vi "Polarisation_v2.vi"(0 "Test Handles Polar":T5, 1 "Polar Params SubVIv2":T2, 3 "Test References":T6) -> (4 "2D Pol Data":dbl[][](array[numeric]), 5 "Test Handles Out":T4, 6 "Angles":dbl[](array[numeric]), 7 "Wavelengths":dbl[](array[numeric]), 8 "Puissances":dbl[](array[numeric]))   [LabVIEW 2019]
uses:
  Light Field/lightfield-automation-labview/LightField Automation.lvclass
  TypeDefs/AcqMode.ctl
  C:/Users/manip/Documents/Controle_Manip_2020/Thorlabs.MotionControl.KCube.SolenoidCLI.dll
  Thorlabs.MotionControl.KCube.SolenoidCLI.dll
  Newport/Newport ESP301/Newport ESP301.lvlib
panel:
  out "Photodiode error out":errorcluster
  out "Photodiode handle out":refnum<visa-resource-name>
  in  "Polar Params SubVI 2":T3
  out "Shutter on?":bool
  in  "Polar mode":u16(ring)=3 caption="Rotate HWP" items=["Excitation"=3, "Detection"=2]
  out "KCube Shutter Device Reference":refnum<k24>
  in  "Previous Button":bool
  in  "StopPolar":bool
  out "CCD 1D Spectrum Main 2":cluster{dbl[], dbl[]}(graph)
  in  "XYGraph Refnum":refnum<vi>
  in  "Acq Mode":T1=enum."Spectrum" caption="Acq mode"
  out "2D Data":dbl[][](array[numeric])
  in  "RotStage Exc Angle (°)":dbl=2.0 caption="Readout (°)" min=-360.0 max=360.0
  out "Position (units)":dbl format="%.6g"
  out "Numeric":i32
  out "Motion Done":bool
  in  "Progress":u8(slide) scale=0.0..100.0
  out "Current angle (°)":dbl
  in  "CCD ROI":T7(ring)
  out "ESP301 Error out":errorcluster
  out "LightField error out":errorcluster
  out "ESP301 Error":errorcluster
  in  "Exposure time (ms)":dbl=100.0
  in  "Axis ESP301 / RotStage":u16(ring) items=["RotStage Detection"=2, "RotStage Excitation"=3]
  in  "Step Angle (°)":dbl=5.0
  in  "End Angle (°)":dbl=180.0
  in  "Start Angle (°)":dbl
  out "LightField Automation out":refnum<class "LightField Automation.lvclass">
  out "VISA resource name out":refnum<visa-resource-name>
types:
  T1 = typedef "AcqMode.ctl" = enum16{"Image", "Spectrum", "APD 1", "APD 2", "APD 1+2"}
  T2 = cluster{"Polar End Angle (°)":dbl, "Polar Start Angle (°)":dbl, "Polar Step Angle (°)":dbl, "Acq Mode":T1, "Polar mode":u16, "Exposure Time (ms)":dbl, "CCD ROI":enum16{"Custom ROI", "Full sensor", "Binned full sensor"}, "KCube Shutter On?":bool}
  T3 = cluster{"Polar End Angle (°)":dbl, "Polar Start Angle (°)":dbl, "Polar Step Angle (°)":dbl, "Acq Mode":T1, "Polar mode":u16, "Exposure Time (ms)":dbl, "CCD ROI":enum16{"Custom ROI", "Full sensor", "Binned full sensor"}}
  T4 = cluster{"LightField Automation out":refnum<class "LightField Automation.lvclass">, "LightField error out":errorcluster, "VISA resource name out":refnum<visa-resource-name>, "ESP301 Error":errorcluster, "Photodiode handle out":refnum<visa-resource-name>, "Photodiode error out":errorcluster}
  T5 = cluster{"LightField Automation out":refnum<class "LightField Automation.lvclass">, "LightField Automation error out":errorcluster, "ESP 301 COM Port":refnum<visa-resource-name>, "ESP 301 Error":errorcluster, "Photodiode handle out":refnum<visa-resource-name>, "Photodiode error out":errorcluster}
  T6 = cluster{"Acquire Polarisation":refnum<vi>, "Save Polarisation":refnum<vi>, "PausePolar":refnum<vi>, "StopPolar":refnum<vi>, "Scan Main Progess Bar":refnum<vi>, "RotStage Exc Angle Readout (°)":refnum<vi>, "RotStage Det Angle Readout (°)":refnum<vi>, "Polarisation 1D Spectrum":refnum<vi>, "Polarisation 2D Image":refnum<vi>, "Shutter Ctrls":refnum<vi>, "KCube Shutter Device Reference":refnum<vi>}
  T7 = enum16{"Custom ROI", "Full sensor", "Binned full sensor"}
  T8 = enum16{"Contrast", "Spectre", "Polarisation", "Time Trace", "XY Intensity Map"}
  T9 = cluster{"Image":dbl[][][], "Frame Size":cluster{"F":i32, "Y":i32, "X":i32}}[]
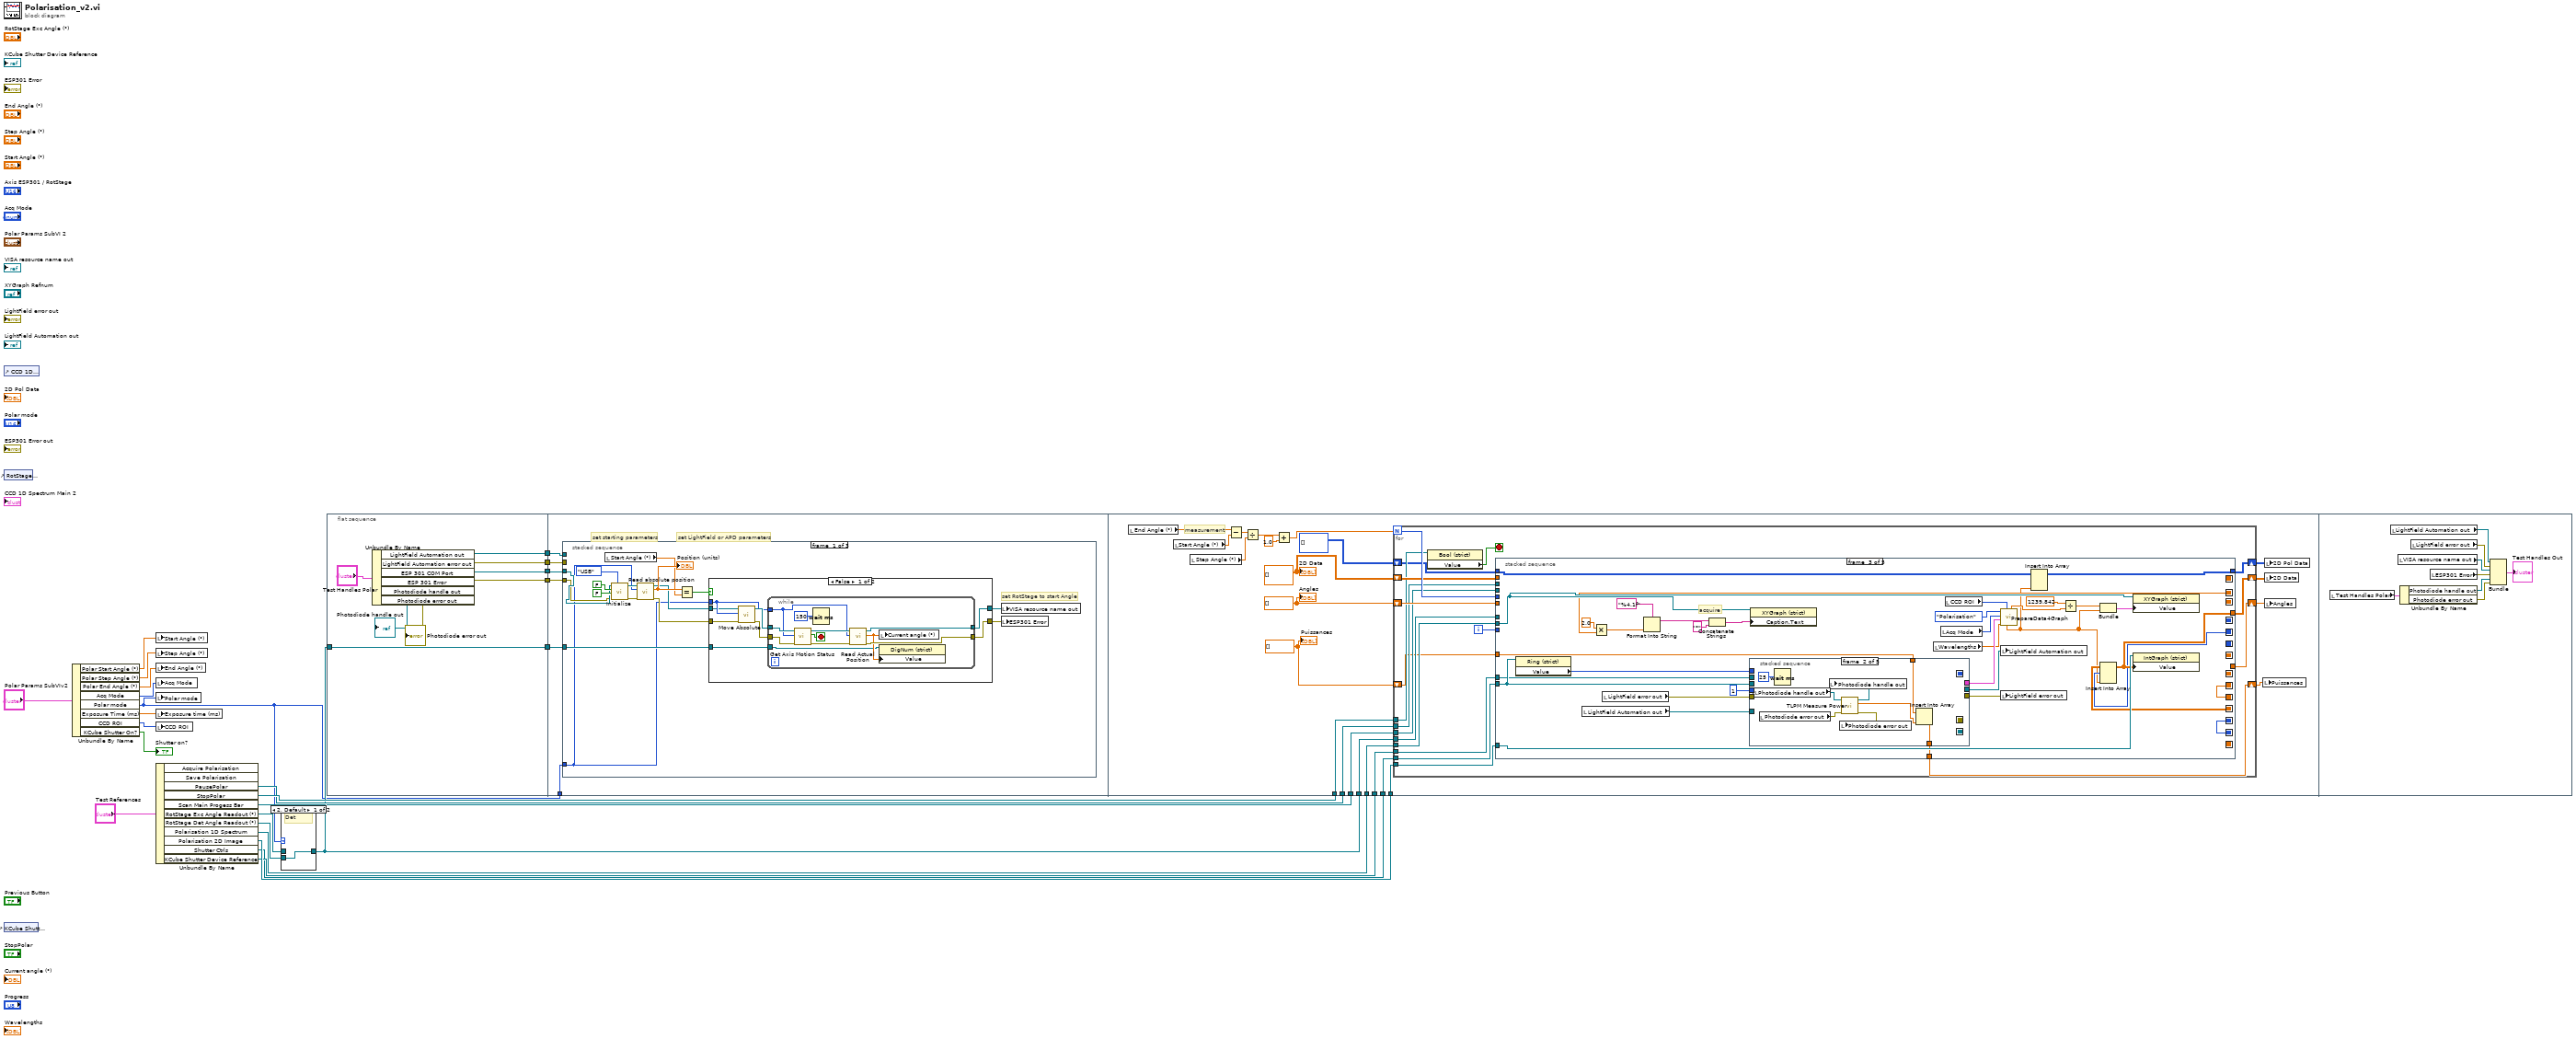
[diagram p0: block diagram]
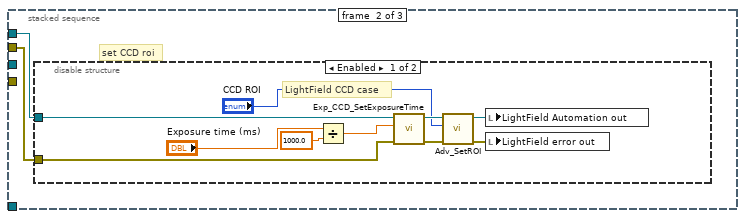
[diagram p4: hidden frame]
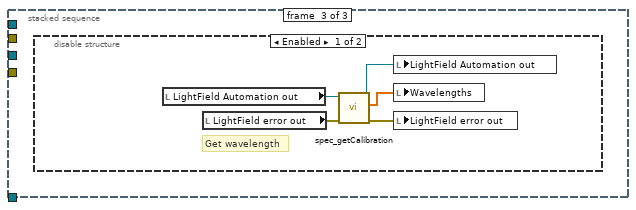
[diagram p6: hidden frame]
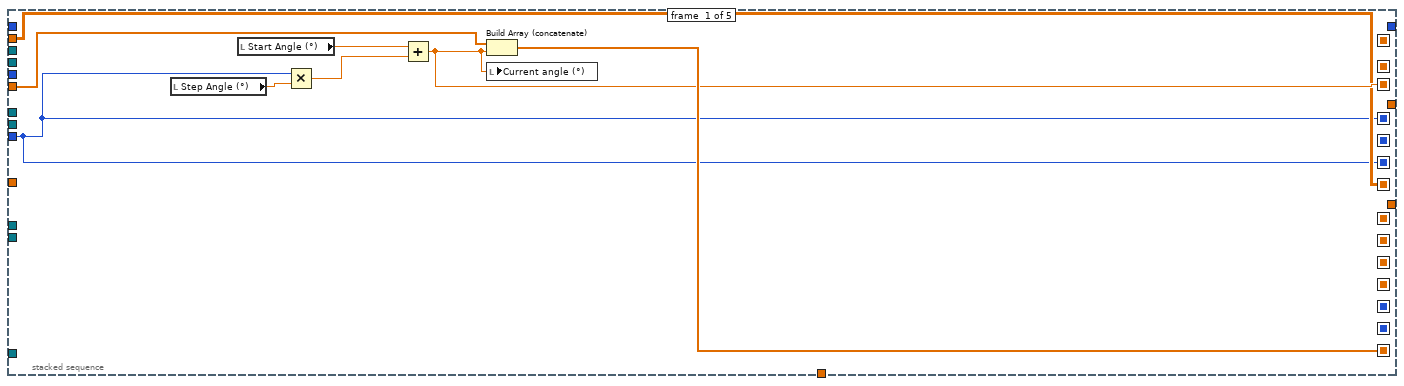
[diagram p8: hidden frame]
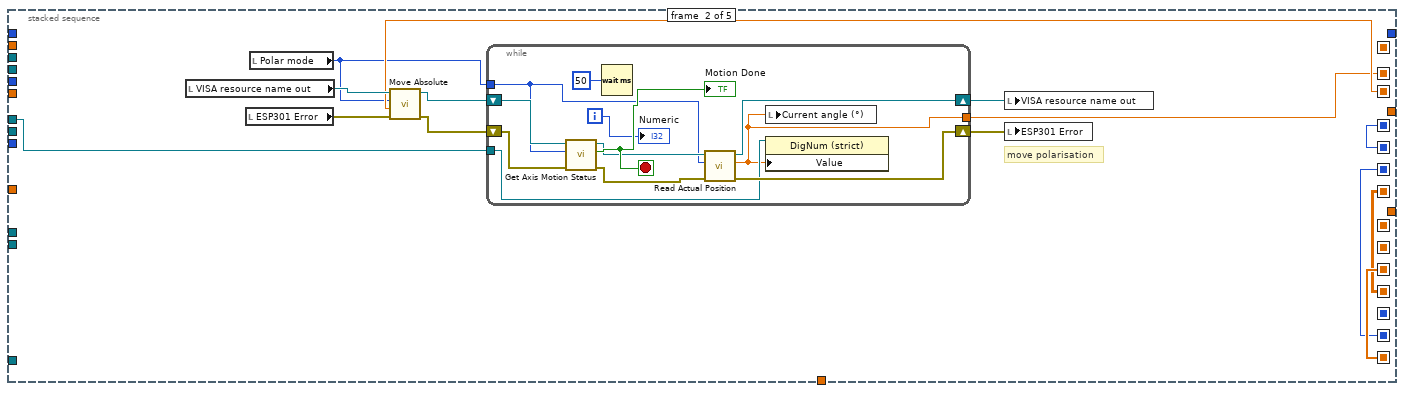
[diagram p9: hidden frame]
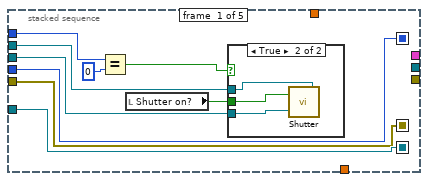
[diagram p10: hidden frame]
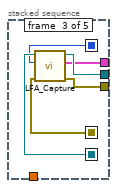
[diagram p12: hidden frame]
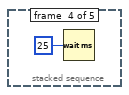
[diagram p13: hidden frame]
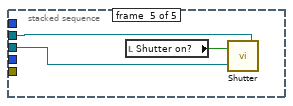
[diagram p14: hidden frame]
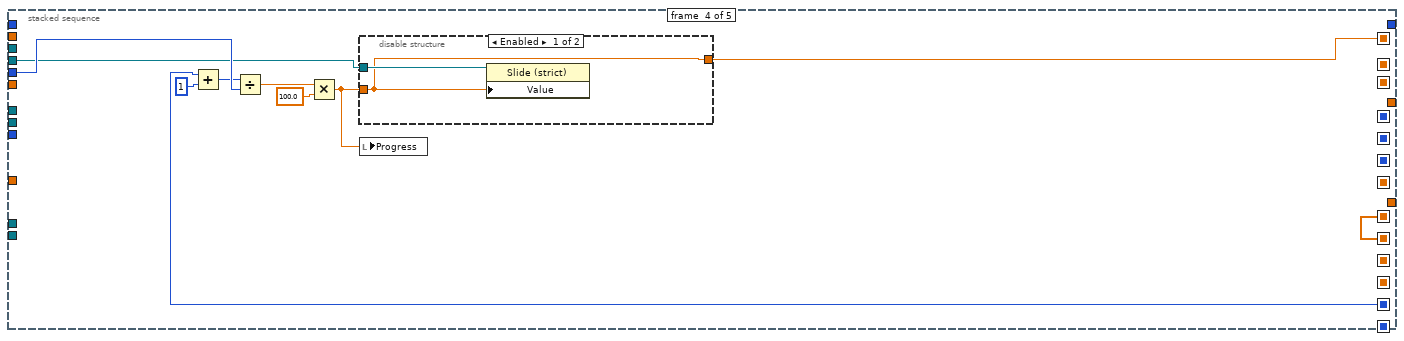
[diagram p15: hidden frame]
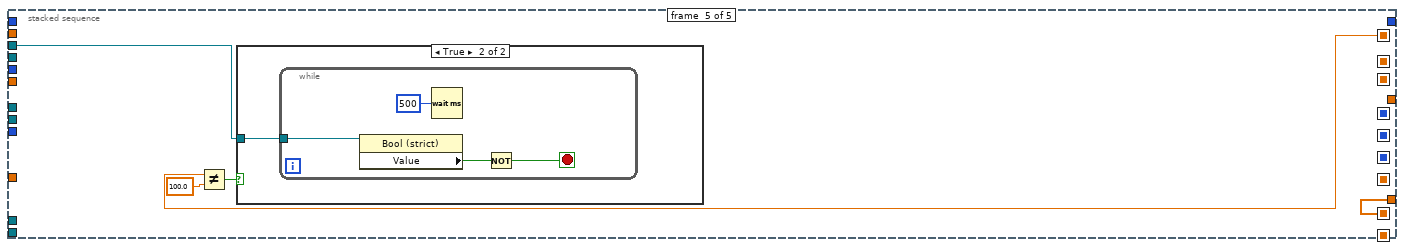
[diagram p17: hidden frame]
diagram:
  n1 = control-ref of="CCD 1D Spectrum Main 2"() -> ()  [unwired: 1 out]
  n2 = control-ref of="RotStage Exc Angle (°)"() -> ()  [unwired: 1 out]
  n3 = control-ref of="KCube Shutter Device Reference"() -> ()  [unwired: 1 out]
  n4 = Unbundle By Name("Polar Params SubVIv2") -> ("Polar Start Angle (°)"=w7:dbl, "Polar Step Angle (°)"=w6:dbl, "Polar End Angle (°)"=w5:dbl, "Acq Mode"=w4:T1, "Polar mode"=w8:u16, "Exposure Time (ms)"=w3:dbl, "CCD ROI"=w2:T7, "KCube Shutter On?"=→"Shutter on?":bool)
  n5 = local write "Start Angle (°)"(w7) -> ()
  n6 = local write "Step Angle (°)"(w6) -> ()
  n7 = local write "End Angle (°)"(w5) -> ()
  n8 = local write "Acq Mode"(w4) -> ()
  n9 = local write "Polar mode"(w8) -> ()
  n10 = local write "Exposure time (ms)"(w3) -> ()
  n11 = local write "CCD ROI"(w2) -> ()
  n12 = Unbundle By Name("Test References") -> ("PausePolar"=w23:refnum<vi>, "StopPolar"=w24:refnum<vi>, "Scan Main Progess Bar"=w17:refnum<vi>, "RotStage Exc Angle Readout (°)"=w18:refnum<vi>, "RotStage Det Angle Readout (°)"=w19:refnum<vi>, "Polarisation 1D Spectrum"=w22:refnum<vi>, "Polarisation 2D Image"=w21:refnum<vi>, "Shutter Ctrls"=w14:refnum<vi>, "KCube Shutter Device Reference"=w15:refnum<vi>)  [unwired: 2 out]
  n13 = case shown="2, Default" w8 {
    tunnel: [w26 w27] -> w20
    tunnel: w19 -> [w26 _]
    tunnel: w18 -> [_ w27]
    frame 2, Default {
      # "Det"
    }
    frame 3 {
      # "Exc"
    }
  }
  n14 = flat-sequence {
    tunnel: w20 -> [w35]
    tunnel: [w35] -> w25
    tunnel: [w33] -> w13
    tunnel: [w32] -> w12
    tunnel: [w31] -> w11
    tunnel: [w30] -> w10
    tunnel: w25 -> [w41]
    tunnel: w13 -> [w40]
    tunnel: w12 -> [w39]
    tunnel: w11 -> [w38]
    tunnel: w10 -> [w37]
    tunnel: w8 -> [w36]
    tunnel: w20 -> [w109]
    tunnel: w21 -> [w108]
    tunnel: w22 -> [w105]
    tunnel: w24 -> [w104]
    tunnel: w23 -> [w103]
    tunnel: w17 -> [w100]
    tunnel: w14 -> [w99]
    tunnel: w15 -> [w98]
    frame #0 {
      n15 = Unbundle By Name("Test Handles Polar") -> ("LightField Automation out"=w31:refnum<class "LightField Automation.lvclass">, "LightField Automation error out"=w30:errorcluster, "ESP 301 COM Port"=w33:refnum<visa-resource-name>, "ESP 301 Error"=w32:errorcluster, "Photodiode handle out"=→"Photodiode handle out":refnum<visa-resource-name>, "Photodiode error out"=→"Photodiode error out":errorcluster)
    }
    frame #1 {
      # "set LightField or APD parameters"
      # "set starting parameters"
      n16 = stacked-sequence {
        tunnel: w41 -> [w45 _ _]
        tunnel: w40 -> [w44 _ _]
        tunnel: w39 -> [w43 _ _]
        tunnel: w38 -> [_ w80 _]
        tunnel: w37 -> [_ w79 _]
        tunnel: w36 -> [w42 _ _]
        frame #0 {
          # "set RotStage to start Angle"
          n17 = local read "Start Angle (°)"() -> (w54:dbl)
          n18 = call "Initialize.vi"("VISA resource name"=w44, "ID Query (True)"=FALSE, "Reset (False)"=FALSE, "error in (no error)"=w43, "Serial Link (RS232)"=enum16{"RS232", "USB"}."USB") -> ("VISA resource name out"=w47:refnum<visa-resource-name>, "error out"=w46:errorcluster)  [unwired: 4 in]
          n19 = call "Read absolute position.vi"("error in (no error)"=w46, "Axis (1)"=w42, "VISA resource name"=w47) -> ("error out"=w52:errorcluster, "Position (units)"=w55:dbl, "VISA resource name out"=w51:refnum<visa-resource-name>)  [unwired: 2 in]
          "Position (units)" <- w55
          n20 = Equal?(x=w55, y=w54) -> (x = y?=w53:bool)
          n21 = case shown="False" w53 {
            tunnel: [w65 w78] -> w57
            tunnel: [w64 w77] -> w56
            tunnel: w42 -> [w61 _]
            tunnel: w52 -> [w60 w77]
            tunnel: w51 -> [w59 w78]
            tunnel: w45 -> [w58 _]
            frame False {
              n22 = call "Move Absolute.vi"("error in (no error)"=w60, "Axis (1)"=w61, "VISA resource name"=w59) -> ("error out"=w62:errorcluster, "VISA resource name out"=w63:refnum<visa-resource-name>)  [unwired: 3 in]
              n23 = while {
                tunnel: w61 -> [w70]
                tunnel: w58 -> [w66]
                tunnel: w63 -> [w76]
                tunnel: [w71] -> w65
                tunnel: w62 -> [w75]
                tunnel: [w68] -> w64
                stop <- w74 stop-if-true
                n24 = call "Get Axis Motion Status.vi"("error in (no error)"=w75, "Axis (1)"=w70, "VISA resource name"=w76) -> ("error out"=w69:errorcluster, "Motion Done"=w74:bool, "VISA resource name out"=w72:refnum<visa-resource-name>)  [unwired: 2 in]
                n25 = Wait (ms)(milliseconds to wait=u32 150) -> ()  [unwired: 1 out]
                n26 = call "Read Actual Position.vi"("error in (no error)"=w69, "Axis (1)"=w70, "VISA resource name"=w72) -> ("error out"=w68:errorcluster, "Position (units)"=w67:dbl, "VISA resource name out"=w71:refnum<visa-resource-name>)  [unwired: 2 in]
                n27 = local write "Current angle (°)"(w67) -> ()
                n28 = property class="DigNum (strict)"(reference=w66, "Value"=w67) -> ()  [unwired: 1 in, 2 out]
              }
            }
            frame True {
            }
          }
          n29 = local write "VISA resource name out"(w57) -> ()
          n30 = local write "ESP301 Error"(w56) -> ()
        }
        frame #1 {
          # "set CCD roi"
          n31 = disable-structure shown="Enabled" {
            disable-tunnel: w80 -> [w82 _]
            disable-tunnel: w79 -> [w81 _]
            frame Enabled {
              # "LightField CCD case"
              n32 = Divide(x="Exposure time (ms)", y=1000.0) -> (x/y=w88:dbl)
              n33 = call "Exp_CCD_SetExposureTime.vi"("error in (no error)"=w81, "Exposure Time (s)"=w88, "LightField Automation in"=w82) -> ("error out"=w86:errorcluster, "LightField Automation out"=w87:refnum<class "LightField Automation.lvclass">)  [unwired: 7 in]
              n34 = call "Adv_SetROI.vi"("error in (no error)"=w86, "ROI"="CCD ROI", "LightField Automation in"=w87) -> ("error out"=w85:errorcluster, "LightField Automation out"=w84:refnum<class "LightField Automation.lvclass">)  [unwired: 7 in]
              n35 = local write "LightField Automation out"(w84) -> ()
              n36 = local write "LightField error out"(w85) -> ()
            }
            frame Disabled {
            }
          }
        }
        frame #2 {
          n37 = disable-structure shown="Enabled" {
            frame Enabled {
              # "Get wavelength"
              n38 = local read "LightField Automation out"() -> (w95:refnum<class "LightField Automation.lvclass">)
              n39 = local read "LightField error out"() -> (w94:errorcluster)
              n40 = call "spec_getCalibration.vi"("error in (no error)"=w94, "LightField Automation in"=w95) -> ("error out"=w92:errorcluster, "ColumnCalibration"=w91:dbl[], "LightField Automation out"=w93:refnum<class "LightField Automation.lvclass">)  [unwired: 7 in]
              n41 = local write "LightField Automation out"(w93) -> ()
              n42 = local write "Wavelengths"(w91) -> ()
              n43 = local write "LightField error out"(w92) -> ()
            }
            frame Disabled {
            }
          }
        }
      }
    }
    frame #2 {
      w97 = dbl[] []
      w107 = dbl[][] []
      w110 = dbl[] []
      # "measurement"
      n44 = local read "End Angle (°)"() -> (w112:dbl)
      n45 = local read "Start Angle (°)"() -> (w113:dbl)
      n46 = local read "Step Angle (°)"() -> (w115:dbl)
      n47 = Subtract(x=w112, y=w113) -> (x-y=w114:dbl)
      n48 = Divide(x=w114, y=w115) -> (x/y=w116:dbl)
      n49 = Add(x=w116, y=1.0) -> (x+y=w117:dbl)
      n50 = for {
        N: w117 -> [w134]
        shift-right: [w136] -> w118
        shift-left: w110 -> [w137]
        tunnel: w100 -> [w133]
        tunnel: w109 -> [w132]
        tunnel: w108 -> [w131]
        shift-right: [w129] -> w106
        shift-left: w107 -> [w130]
        tunnel: w105 -> [w128]
        tunnel: w104 -> [w127]
        tunnel: w103 -> [w125]
        shift-right: [w123] -> w101
        shift-left: i32[][] [] -> [w124]
        tunnel: w99 -> [w122]
        tunnel: w98 -> [w121]
        shift-right: [w119] -> w96
        shift-left: w97 -> [w120]
        i -> [w135]
        stop <- w126 stop-if-true
        n51 = property class="Bool (strict)"(reference=w127) -> ("Value"=w126:bool)  [unwired: 1 in, 2 out]
        n52 = stacked-sequence {
          seq-local: [w144 _ _ _ _] -> [_ w159 _ _ _]
          seq-local: [w138 _ _ _ _] -> [_ w158 _ _ _]
          seq-local: [w140 _ _ _ _] -> [_ w155 _ _ _]
          seq-local: [w139 _ _ _ _] -> [_ w148 _ _ _]
          seq-local: [w138 _ _ _ _] -> [_ w147 _ _ _]
          seq-local: [_ w159 _ _ _] -> [_ _ w204 _ _]
          seq-local: [_ w158 _ _ _] -> [_ _ w207 _ _]
          seq-local: [_ w148 _ _ _] -> [_ _ w205 _ _]
          seq-local: [_ w147 _ _ _] -> [_ _ w202 _ _]
          seq-local: [_ w146 _ _ _] -> [_ _ w183 _ _]
          seq-local: [_ _ w204 _ _] -> [_ _ _ w247 _]
          seq-local: [_ _ w207 _ _] -> [_ _ _ w243 _]
          seq-local: [_ _ _ w247 _] -> [_ _ _ _ w254]
          seq-local: [_ _ _ w238 _] -> [_ _ _ _ w252]
          tunnel: w137 -> [w145 _ _ _ _]
          tunnel: w135 -> [w138 _ _ _ _]
          tunnel: w130 -> [w139 _ _ _ _]
          tunnel: w132 -> [_ w149 _ _ _]
          tunnel: w131 -> [_ _ w206 _ _]
          tunnel: [_ _ w203 _ _] -> w129
          tunnel: w128 -> [_ _ w193 _ _]
          tunnel: w124 -> [_ _ w181 _ _]
          tunnel: [_ _ w180 _ _] -> w123
          tunnel: w122 -> [_ _ w175 _ _]
          tunnel: w121 -> [_ _ w174 _ _]
          tunnel: w134 -> [_ _ _ w244 _]
          tunnel: w133 -> [_ _ _ w240 _]
          tunnel: [_ _ _ _ w254] -> w136
          tunnel: w125 -> [_ _ _ _ w253]
          tunnel: w120 -> [_ _ w173 _ _]
          tunnel: [_ _ w172 _ _] -> w119
          frame #0 {
            n53 = local read "Step Angle (°)"() -> (w142:dbl)
            n54 = local read "Start Angle (°)"() -> (w143:dbl)
            n55 = Multiply(x=w138, y=w142) -> (x*y=w141:dbl)
            n56 = Add(x=w143, y=w141) -> (x+y=w140:dbl)
            n57 = Build Array (concatenate)(w145, w140) -> (w144:dbl[])
            n58 = local write "Current angle (°)"(w140) -> ()
          }
          frame #1 {
            # "move polarisation"
            n59 = local read "VISA resource name out"() -> (w157:refnum<visa-resource-name>)
            n60 = local read "ESP301 Error"() -> (w156:errorcluster)
            n61 = local read "Polar mode"() -> (w152:u16)
            n62 = call "Move Absolute.vi"("error in (no error)"=w156, "Position (0 units)"=w155, "Axis (1)"=w152, "VISA resource name"=w157) -> ("error out"=w154:errorcluster, "VISA resource name out"=w153:refnum<visa-resource-name>)  [unwired: 2 in]
            n63 = while {
              tunnel: w152 -> [w164]
              shift-right: [w163] -> w150
              shift-left: w153 -> [w169]
              shift-right: [w162] -> w151
              shift-left: w154 -> [w170]
              tunnel: w149 -> [w161]
              tunnel: [w160] -> w146
              i -> [w168]
              stop <- w171 stop-if-true
              n64 = call "Get Axis Motion Status.vi"("error in (no error)"=w170, "Axis (1)"=w164, "VISA resource name"=w169) -> ("error out"=w166:errorcluster, "Motion Done"=w171:bool, "VISA resource name out"=w165:refnum<visa-resource-name>)  [unwired: 2 in]
              "Motion Done" <- w171
              n65 = Wait (ms)(milliseconds to wait=u32 50) -> ()  [unwired: 1 out]
              n66 = call "Read Actual Position.vi"("error in (no error)"=w166, "Axis (1)"=w164, "VISA resource name"=w165) -> ("error out"=w162:errorcluster, "Position (units)"=w160:dbl, "VISA resource name out"=w163:refnum<visa-resource-name>)  [unwired: 2 in]
              n67 = local write "Current angle (°)"(w160) -> ()
              n68 = property class="DigNum (strict)"(reference=w161, "Value"=w160) -> ()  [unwired: 1 in, 2 out]
              "Numeric" <- w168
            }
            n69 = local write "VISA resource name out"(w150) -> ()
            n70 = local write "ESP301 Error"(w151) -> ()
          }
          frame #2 {
            # "acquire"
            n71 = property class="Ring (strict)"(reference=w175) -> ("Value"=w182:u16)  [unwired: 1 in, 2 out]
            n72 = local read "LightField Automation out"() -> (w201:refnum<class "LightField Automation.lvclass">)
            n73 = Multiply(x=2.0, y=w183) -> (x*y=w185:dbl)
            n74 = local read "LightField error out"() -> (w200:errorcluster)
            n75 = Format Into String(format string="%4.1f", w185) -> (resulting string=w192:string)  [unwired: 2 in, 1 out]
            n76 = Concatenate Strings(w192, "°") -> (w190:string)
            n77 = stacked-sequence {
              seq-local: [w216 _ _ _ _] -> [_ _ w233 _ _]
              seq-local: [w215 _ _ _ _] -> [_ _ w232 _ _]
              seq-local: [w214 _ _ _ _] -> [_ _ w228 _ _]
              tunnel: w201 -> [w216 _ _ _ _]
              tunnel: w200 -> [w215 _ _ _ _]
              tunnel: 1 ("Frames") -> [w214 _ _ _ _]
              tunnel: [_ _ w231 _ _] -> w199
              tunnel: [_ _ w230 _ _] -> w198
              tunnel: [_ _ w229 _ _] -> w197
              tunnel: w175 -> [w212 _ _ _ w237]
              tunnel: w174 -> [w213 _ _ _ w236]
              tunnel: w182 -> [w211 _ _ _ _]
              tunnel: w173 -> [_ w222 _ _ _]
              tunnel: [_ w220 _ _ _] -> w172
              frame #0 {
                n78 = Equal?(x=w211, y=u16 0) -> (x = y?=w210:bool)
                n79 = local read "Shutter on?"() -> (w208:bool)
                n80 = case shown="True" w210 {
                  tunnel: w213 -> [_ w219]
                  tunnel: w212 -> [_ w218]
                  tunnel: w208 -> [_ w217]
                  frame False {
                  }
                  frame True {
                    n81 = call "Shutter.vi"("KCube Shutter Device Reference 2"=w219, "Shutter Ctrls 2"=w218, "Shutter on?"=w217) -> ()
                  }
                }
              }
              frame #1 {
                n82 = local read "Photodiode handle out"() -> (w226:refnum<visa-resource-name>)
                n83 = local read "Photodiode error out"() -> (w225:errorcluster)
                n84 = Wait (ms)(milliseconds to wait=u32 25) -> ()  [unwired: 1 out]
                n85 = call <instrlib>:"TLPM Measure Power.vi"("error in (no error)"=w225, "instrument handle"=w226) -> ("error out"=w223:errorcluster, "Power"=w221:dbl, "instrument handle out"=w224:refnum<visa-resource-name>)  [unwired: 7 in]
                n86 = local write "Photodiode handle out"(w224) -> ()
                n87 = local write "Photodiode error out"(w223) -> ()
                n88 = Insert Into Array(array=w222, new element=w221) -> (w220:dbl[])  [unwired: 1 in]
              }
              frame #2 {
                n89 = call "LFA_Capture.vi"("error in (no error)"=w232, "Frames"=w228, "LightField Automation in"=w233) -> ("error out"=w231:errorcluster, "Data"=w229:T9, "LightField Automation out"=w230:refnum<class "LightField Automation.lvclass">)  [unwired: 6 in]
              }
              frame #3 {
                n90 = Wait (ms)(milliseconds to wait=u32 25) -> ()  [unwired: 1 out]
              }
              frame #4 {
                n91 = local read "Shutter on?"() -> (w235:bool)
                n92 = call "Shutter.vi"("KCube Shutter Device Reference 2"=w236, "Shutter Ctrls 2"=w237, "Shutter on?"=w235) -> ()
              }
            }
            n93 = property class="XYGraph (strict)"(reference=w193, "Caption.Text"=w190) -> ()  [unwired: 1 in, 2 out]
            n94 = local read "Wavelengths"() -> (w194:dbl[])
            n95 = local read "Acq Mode"() -> (w195:T1)
            n96 = local read "CCD ROI"() -> (w176:T7)
            n97 = call "PrepareData4Graph.vi"("Wavelength nm"=w194, "DataLF"=w197, "CCD ROI"=w176, "AcqMode"=w195, "Data type"=T8."Polarisation") -> ("Wavelength out"=w179:dbl[], "PLInt out"=w178:dbl[])  [unwired: 1 in, 3 out]
            n98 = local write "LightField Automation out"(w198) -> ()
            n99 = local write "LightField error out"(w199) -> ()
            n100 = Insert Into Array(array=w181, new element=w178) -> (w180:i32[][])  [unwired: 2 in]
            n101 = Divide(x=1239.842, y=w179) -> (x/y=w186:dbl[])
            n102 = Bundle(w186, "PLInt out"=w178) -> (w187:cluster{dbl[], "PLInt out":dbl[]})  [unwired: 1 in]
            n103 = Insert Into Array(array=w205, index (row)=w202, new element=w178) -> (w203:dbl[][])  [unwired: 1 in]
            n104 = property class="XYGraph (strict)"(reference=w193, "Value"=w187) -> ()  [unwired: 1 in, 2 out]
            n105 = property class="IntGraph (strict)"(reference=w206, "Value"=w203) -> ()  [unwired: 1 in, 2 out]
          }
          frame #3 {
            n106 = Add(x=w243, y=1) -> (x+y=w241:i32)
            n107 = Divide(x=w241, y=w244) -> (x/y=w246:dbl)
            n108 = Multiply(x=w246, y=100.0) -> (x*y=w239:dbl)
            n109 = disable-structure shown="Enabled" {
              disable-tunnel: w240 -> [w249 _]
              disable-tunnel: w239 -> [w248 _]
              disable-tunnel: [w248 _] -> w238
              frame Enabled {
                n110 = property class="Slide (strict)"(reference=w249, "Value"=w248) -> ()  [unwired: 1 in, 2 out]
              }
              frame Disabled {
              }
            }
            n111 = local write "Progress"(w239) -> ()
          }
          frame #4 {
            n112 = Not Equal?(x=w252, y=100.0) -> (x != y?=w250:bool)
            n113 = case shown="True" w250 {
              tunnel: w253 -> [_ w255]
              frame False {
              }
              frame True {
                n114 = while {
                  tunnel: w255 -> [w258]
                  stop <- w256 stop-if-true
                  n115 = property class="Bool (strict)"(reference=w258) -> ("Value"=w257:bool)  [unwired: 1 in, 2 out]
                  n116 = Wait (ms)(milliseconds to wait=u32 500) -> ()  [unwired: 1 out]
                  n117 = Not(x=w257) -> (.not. x?=w256:bool)
                }
              }
            }
          }
        }
      }
      n118 = local write "Puissances"(w96) -> ()
      n119 = local write "2D Pol Data"(w101) -> ()
      n120 = local write "2D Data"(w106) -> ()
      n121 = local write "Angles"(w118) -> ()
      "Angles" <- w110
      "2D Data" <- w107
      "Puissances" <- w97
    }
    frame #3 {
      n122 = local read "Test Handles Polar"() -> (w263:T5)
      n123 = local read "LightField Automation out"() -> (w267:refnum<class "LightField Automation.lvclass">)
      n124 = local read "VISA resource name out"() -> (w265:refnum<visa-resource-name>)
      n125 = Unbundle By Name(w263) -> ("Photodiode handle out"=w262:refnum<visa-resource-name>, "Photodiode error out"=w261:errorcluster)
      n126 = local read "LightField error out"() -> (w266:errorcluster)
      n127 = local read "ESP301 Error"() -> (w264:errorcluster)
      n128 = Bundle("LightField Automation out"=w267, "LightField error out"=w266, "VISA resource name out"=w265, "ESP301 Error"=w264, "Photodiode handle out"=w262, "Photodiode error out"=w261) -> (→"Test Handles Out":T4)  [unwired: 1 in]
    }
  }
